vi "Smoothie Comm.vi"(11 "INITIALISE":bool) -> ()   [LabVIEW 2016]
uses:
  <vilib>/Instr/_visa.llb/VISA Open Access Mode.ctl
panel:
  in  "SMOOTHIE VISA IN":refnum<visa-resource-name>
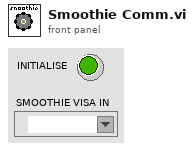
[diagram p1: front panel]
types:
  T1 = typedef "VISA Open Access Mode.ctl" = u32
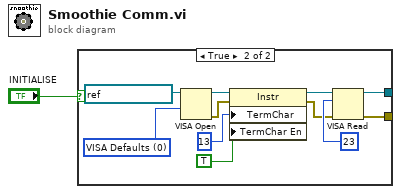
[diagram p0: block diagram]
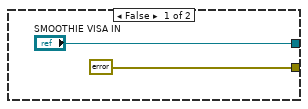
[diagram p2: hidden frame]
diagram:
  n1 = case shown="True" "INITIALISE" {
    tunnel: ["SMOOTHIE VISA IN" w5] -> _
    tunnel: [errorcluster {"status"=FALSE, "code"=0, "source"=""} ("error out") w4] -> _
    frame False {
    }
    frame True {
      w8 = T1 0 items=["VISA Defaults"=0, "Exclusive Lock"=1, "Load Configured Settings"=4] ("Access Mode")
      n2 = VISA Open(access mode=w8, VISA resource name=refnum<visa-resource-name> "SMOOTHIE") -> (VISA resource name=w10:refnum<visa-resource-name>, error out=w9:errorcluster)  [unwired: 3 in]
      n3 = property class="Instr"(reference=w10, error in=w9, "TermChar"=u8 13 ("Message Based Settings:Termination Character"), "TermChar En"=TRUE ("Message Based Settings:Termination Character Enable")) -> (reference out=w7:refnum<visa-resource-name>, error out=w6:errorcluster)
      n4 = VISA Read(VISA resource name=w7, byte count=u32 23, error in (no error)=w6) -> (VISA resource name out=w5:refnum<visa-resource-name>, error out=w4:errorcluster)  [unwired: 2 out]
    }
  }
